vi "PLCtest.vi"(7 "Old VAL":bool[](array[boolean]), 10 "索引":i32, 11 "VISA资源名称":refnum<visa-resource-name>="COM2") -> (0 "错误输出":errorcluster)   [LabVIEW 2011]
uses:
  <vilib>/Instr/_visa.llb/VISA Configure Serial Port (Instr).vi
panel:
  in  "错误输入（无错误） 2":errorcluster caption="错误输入（无错误）"
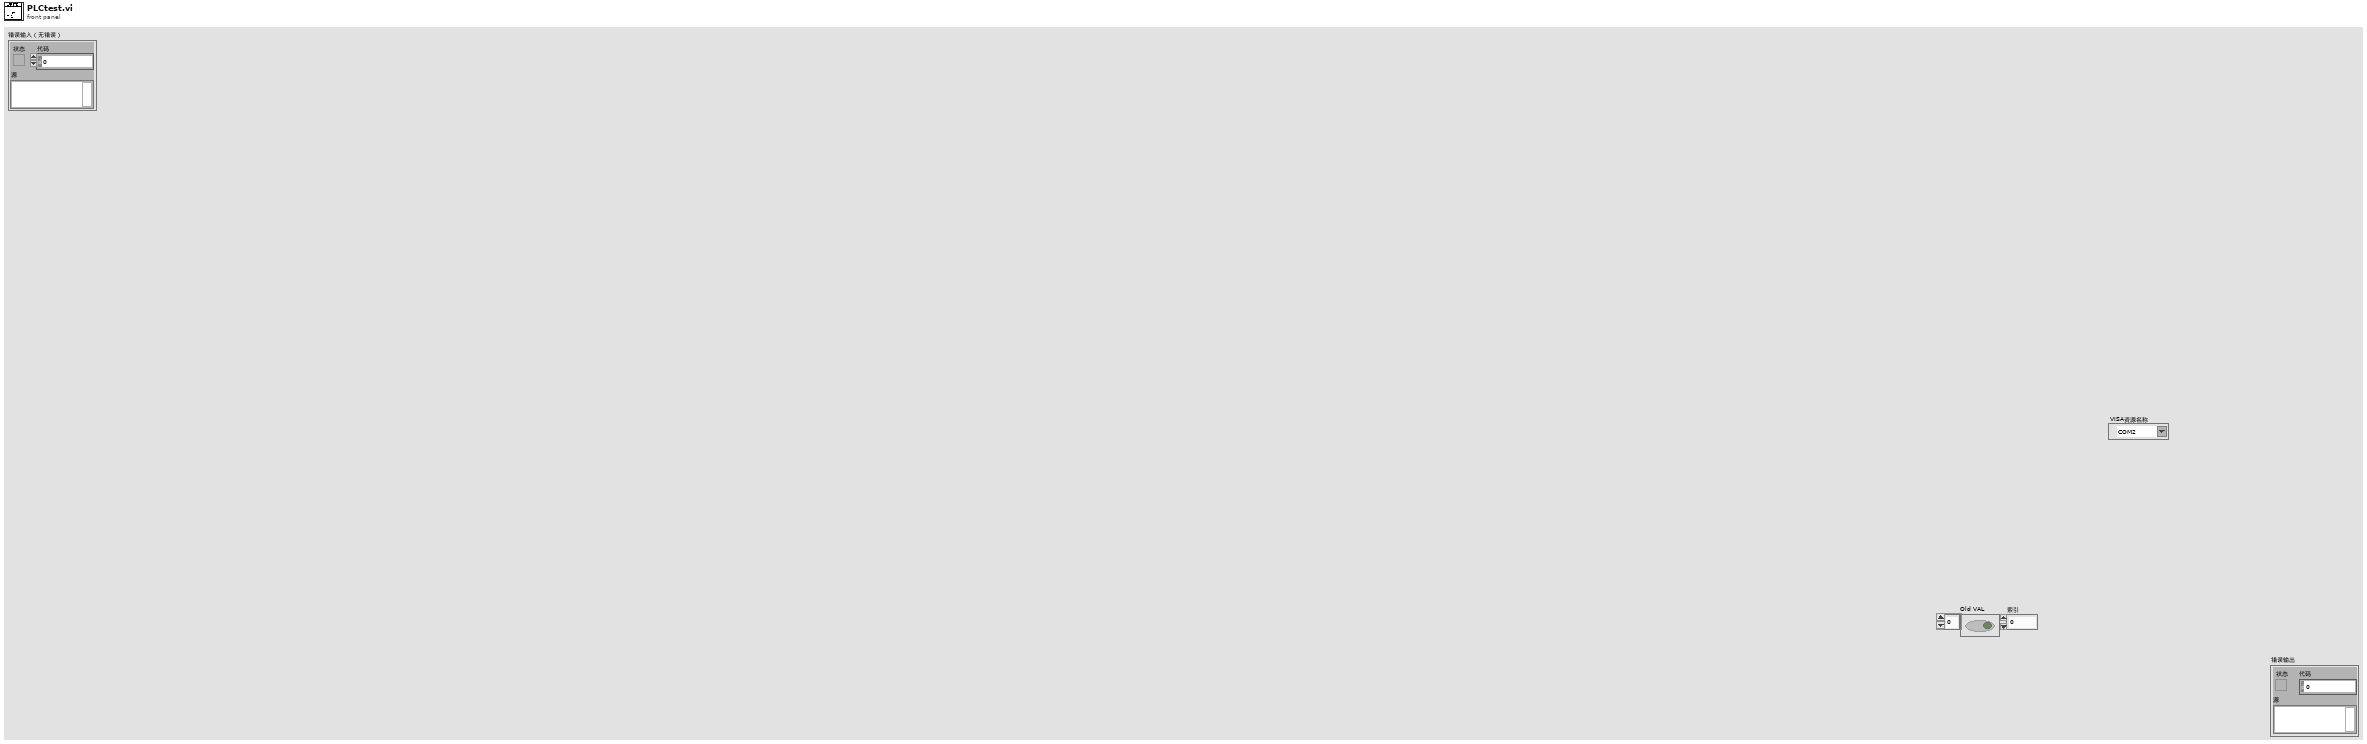
[diagram p1: front panel]
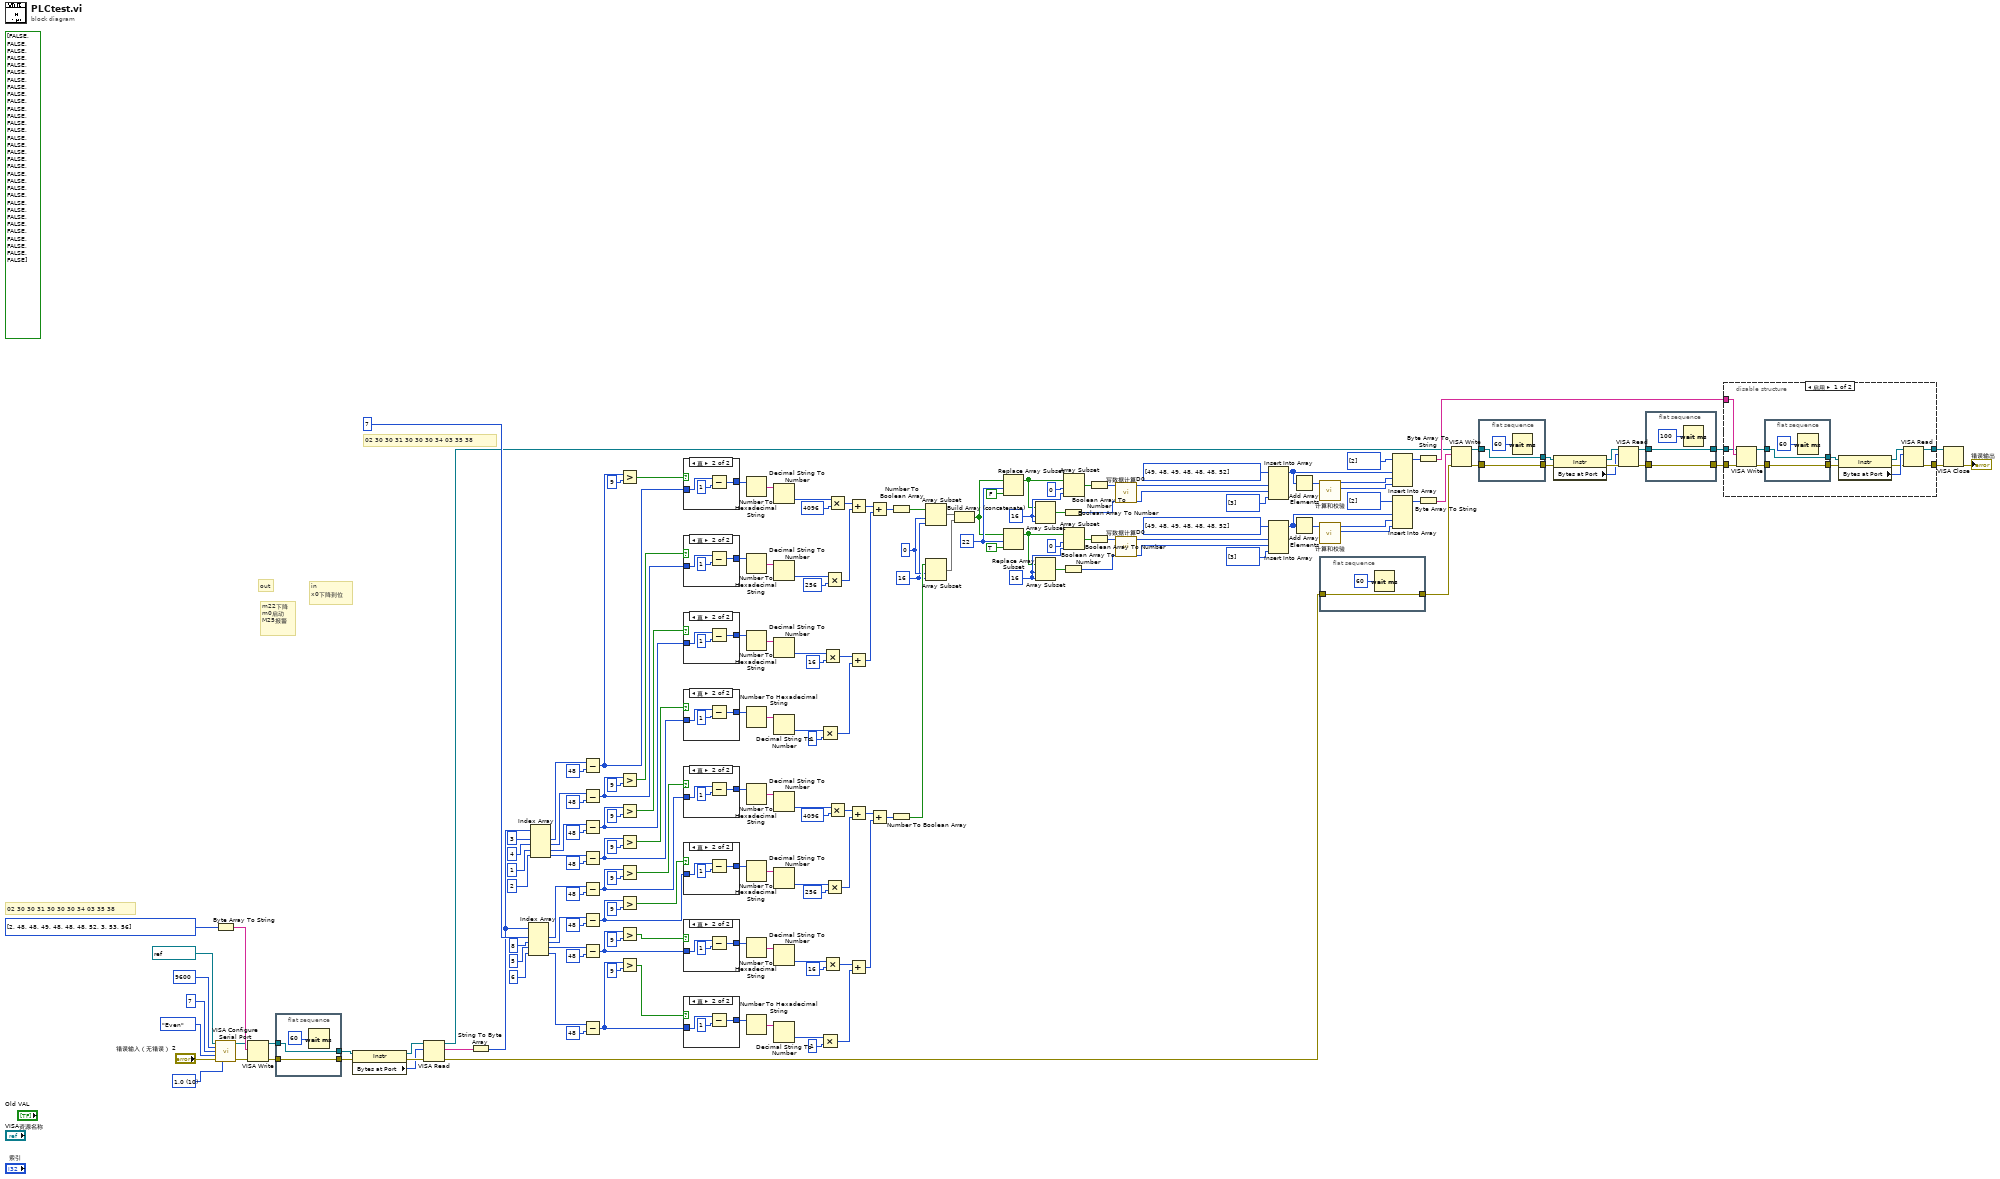
[diagram p0: block diagram]
diagram:
  w10 = u16 10 items=["1.0"=10, "1.5"=15, "2.0"=20] ("停止位")
  w15 = 16 ("长度")
  w16 = 0 ("索引")
  (unwired) bool[] [FALSE, FALSE, FALSE, FALSE, FALSE, FALSE, FALSE, FALSE, FALSE, FALSE, FALSE, FALSE, FALSE, FALSE, FALSE, FALSE, FALSE, FALSE, FALSE, FALSE, FALSE, FALSE, FALSE, FALSE, FALSE, FALSE, FALSE, FALSE, FALSE, FALSE, FALSE, FALSE] ("M 2")
  w124 = 22 ("索引")
  w149 = 16 ("长度")
  w155 = 16 ("长度")
  # "in\nx0下降到位"
  # "out"
  # "02 30 30 31 30 30 30 34 03 35 38"
  # "02 30 30 31 30 30 30 34 03 35 38"
  # "m22下降\nm0启动\nM25报警"
  n1 = Byte Array To String(unsigned byte array=u8[] [2, 48, 48, 49, 48, 48, 48, 52, 3, 53, 56] ("无符号字节数组")) -> (string=w121:string)
  n2 = call-poly "VISA Configure Serial Port"("VISA resource name"=refnum<visa-resource-name> "COM2" ("VISA资源名称"), "baud rate (9600)"=u32 9600 ("波特率"), "data bits (8)"=u16 7 ("数据位"), "parity (0:none)"=enum16{"None", "Odd", "Even", "Mark", "Space"}."Even" ("校验位"), "error in (no error)"="错误输入（无错误） 2", "stop bits (10: 1 bit)"=w10) -> ("VISA resource name out"=w5:refnum<visa-resource-name>, "error out"=w3:errorcluster)  [unwired: 8 in]
  n3 = VISA Write(VISA resource name=w5, write buffer=w121, error in (no error)=w3) -> (VISA resource name out=w122:refnum<visa-resource-name>, error out=w123:errorcluster)  [unwired: 1 out]
  n4 = flat-sequence {
    tunnel: w123 -> [w179]
    tunnel: [w179] -> w116
    tunnel: w122 -> [w178]
    tunnel: [w178] -> w117
    frame #0 {
      n5 = Wait (ms)(milliseconds to wait=u32 60 ("等待时间（毫秒）")) -> ()  [unwired: 1 out]
    }
  }
  n6 = property class="Instr"(reference=w117, error in=w116) -> (reference out=w120:refnum<visa-resource-name>, error out=w119:errorcluster, "Bytes at Port"=w118:u32)
  n7 = VISA Read(VISA resource name=w120, byte count=w118, error in (no error)=w119) -> (VISA resource name out=w11:refnum<visa-resource-name>, read buffer=w115:string, error out=w2:errorcluster)  [unwired: 1 out]
  n8 = String To Byte Array(string=w115) -> (unsigned byte array=w20:u8[])
  n9 = Index Array(array=w20, index #1=7 ("索引"), index #2=8 ("索引"), index #3=5 ("索引"), index #4=6 ("索引")) -> (element #1=w25:u8, element #2=w28:u8, element #3=w30:u8, element #4=w32:u8)
  n10 = Index Array(array=w20, index #1=3 ("索引"), index #2=4 ("索引"), index #3=1 ("索引"), index #4=2 ("索引")) -> (element #1=w110:u8, element #2=w107:u8, element #3=w105:u8, element #4=w103:u8)
  n11 = Subtract(x=w110, y=u8 48) -> (x-y=w91:u8)
  n12 = Subtract(x=w107, y=u8 48) -> (x-y=w94:u8)
  n13 = Subtract(x=w105, y=u8 48) -> (x-y=w97:u8)
  n14 = Subtract(x=w103, y=u8 48) -> (x-y=w101:u8)
  n15 = Subtract(x=w25, y=u8 48) -> (x-y=w44:u8)
  n16 = Subtract(x=w28, y=u8 48) -> (x-y=w41:u8)
  n17 = Subtract(x=w30, y=u8 48) -> (x-y=w38:u8)
  n18 = Subtract(x=w32, y=u8 48) -> (x-y=w34:u8)
  n19 = Greater?(x=w91, y=u8 9) -> (0:w93:bool)
  n20 = Greater?(x=w94, y=u8 9) -> (0:w95:bool)
  n21 = Greater?(x=w97, y=u8 9) -> (0:w99:bool)
  n22 = Greater?(x=w101, y=u8 9) -> (0:w100:bool)
  n23 = Greater?(x=w44, y=u8 9) -> (0:w42:bool)
  n24 = Greater?(x=w41, y=u8 9) -> (0:w40:bool)
  n25 = Greater?(x=w38, y=u8 9) -> (0:w36:bool)
  n26 = Greater?(x=w34, y=u8 9) -> (0:w35:bool)
  n27 = case shown="真" w93 {
    tunnel: w91 -> [w180 w183]
    tunnel: [w180 w181] -> w90
    frame False {
    }
    frame True {
      n28 = Subtract(x=w183, y=u8 1) -> (x-y=w181:u8)
    }
  }
  n29 = case shown="真" w95 {
    tunnel: w94 -> [w184 w187]
    tunnel: [w184 w185] -> w89
    frame False {
    }
    frame True {
      n30 = Subtract(x=w187, y=u8 1) -> (x-y=w185:u8)
    }
  }
  n31 = case shown="真" w99 {
    tunnel: w97 -> [w188 w191]
    tunnel: [w188 w189] -> w88
    frame False {
    }
    frame True {
      n32 = Subtract(x=w191, y=u8 1) -> (x-y=w189:u8)
    }
  }
  n33 = case shown="真" w100 {
    tunnel: w101 -> [w192 w195]
    tunnel: [w192 w193] -> w87
    frame False {
    }
    frame True {
      n34 = Subtract(x=w195, y=u8 1) -> (x-y=w193:u8)
    }
  }
  n35 = case shown="真" w42 {
    tunnel: w44 -> [w196 w199]
    tunnel: [w196 w197] -> w45
    frame False {
    }
    frame True {
      n36 = Subtract(x=w199, y=u8 1) -> (x-y=w197:u8)
    }
  }
  n37 = case shown="真" w40 {
    tunnel: w41 -> [w200 w203]
    tunnel: [w200 w201] -> w46
    frame False {
    }
    frame True {
      n38 = Subtract(x=w203, y=u8 1) -> (x-y=w201:u8)
    }
  }
  n39 = case shown="真" w36 {
    tunnel: w38 -> [w204 w207]
    tunnel: [w204 w205] -> w47
    frame False {
    }
    frame True {
      n40 = Subtract(x=w207, y=u8 1) -> (x-y=w205:u8)
    }
  }
  n41 = case shown="真" w35 {
    tunnel: w34 -> [w208 w211]
    tunnel: [w208 w209] -> w48
    frame False {
    }
    frame True {
      n42 = Subtract(x=w211, y=u8 1) -> (x-y=w209:u8)
    }
  }
  n43 = Number To Hexadecimal String(2:w90) -> (0:w86:string)  [unwired: 1 in]
  n44 = Number To Hexadecimal String(2:w89) -> (0:w85:string)  [unwired: 1 in]
  n45 = Number To Hexadecimal String(2:w88) -> (0:w84:string)  [unwired: 1 in]
  n46 = Number To Hexadecimal String(2:w87) -> (0:w83:string)  [unwired: 1 in]
  n47 = Number To Hexadecimal String(2:w45) -> (0:w49:string)  [unwired: 1 in]
  n48 = Number To Hexadecimal String(2:w46) -> (0:w50:string)  [unwired: 1 in]
  n49 = Number To Hexadecimal String(2:w47) -> (0:w51:string)  [unwired: 1 in]
  n50 = Number To Hexadecimal String(2:w48) -> (0:w52:string)  [unwired: 1 in]
  n51 = Decimal String To Number(string=w86) -> (number=w82:i32)  [unwired: 2 in, 1 out]
  n52 = Decimal String To Number(string=w85) -> (number=w81:i32)  [unwired: 2 in, 1 out]
  n53 = Decimal String To Number(string=w84) -> (number=w80:i32)  [unwired: 2 in, 1 out]
  n54 = Decimal String To Number(string=w83) -> (number=w79:i32)  [unwired: 2 in, 1 out]
  n55 = Decimal String To Number(string=w49) -> (number=w53:i32)  [unwired: 2 in, 1 out]
  n56 = Decimal String To Number(string=w50) -> (number=w54:i32)  [unwired: 2 in, 1 out]
  n57 = Decimal String To Number(string=w51) -> (number=w55:i32)  [unwired: 2 in, 1 out]
  n58 = Decimal String To Number(string=w52) -> (number=w56:i32)  [unwired: 2 in, 1 out]
  n59 = Multiply(x=w79, y=1) -> (x*y=w73:i32)
  n60 = Multiply(x=w56, y=1) -> (x*y=w62:i32)
  n61 = Multiply(x=w80, y=16) -> (x*y=w72:i32)
  n62 = Multiply(x=w55, y=16) -> (x*y=w63:i32)
  n63 = Multiply(x=w81, y=256) -> (x*y=w74:i32)
  n64 = Multiply(x=w54, y=256) -> (x*y=w61:i32)
  n65 = Multiply(x=w82, y=4096) -> (x*y=w69:i32)
  n66 = Multiply(x=w53, y=4096) -> (x*y=w66:i32)
  n67 = Add(x=w69, y=w74) -> (x+y=w70:i32)
  n68 = Add(x=w72, y=w73) -> (x+y=w71:i32)
  n69 = Add(x=w66, y=w61) -> (x+y=w65:i32)
  n70 = Add(x=w63, y=w62) -> (x+y=w64:i32)
  n71 = Add(x=w70, y=w71) -> (x+y=w68:i32)
  n72 = Add(x=w65, y=w64) -> (x+y=w67:i32)
  n73 = Number To Boolean Array(number=w68) -> (Boolean array=w17:bool[])
  n74 = Number To Boolean Array(number=w67) -> (Boolean array=w18:bool[])
  n75 = Array Subset(array=w17, index=w16, length=w15) -> (w13:bool[])
  n76 = Array Subset(array=w18, index=w16, length=w15) -> (w14:bool[])
  n77 = Build Array (concatenate)(w13, w14) -> (w12:bool[])
  n78 = Replace Array Subset(array=w12, new element=FALSE, index=w124) -> (w128:bool[])
  n79 = Replace Array Subset(array=w12, new element=TRUE ("Val"), index=w124) -> (w154:bool[])
  n80 = Array Subset(array=w128, index=w149, length=w149) -> (w151:bool[])
  n81 = Array Subset(array=w154, index=w155, length=w155) -> (w152:bool[])
  n82 = Boolean Array To Number(Boolean array=w151) -> (number=w147:u32)
  n83 = Boolean Array To Number(Boolean array=w152) -> (number=w157:u32)
  n84 = Array Subset(array=w128, index=0 ("索引"), length=w149) -> (w150:bool[])
  n85 = Array Subset(array=w154, index=0 ("索引"), length=w155) -> (w153:bool[])
  n86 = Boolean Array To Number(Boolean array=w150) -> (number=w146:u32)
  n87 = Boolean Array To Number(Boolean array=w153) -> (number=w158:u32)
  n88 = call "写数据计算D0.vi"("D0 2"=w147, "D0"=w146) -> ("数组 2"=w145:u32[], "数组"=w139:u32[])  [unwired: 8 in]
  n89 = call "写数据计算D0.vi"("D0 2"=w157, "D0"=w158) -> ("数组 2"=w159:u32[], "数组"=w165:u32[])  [unwired: 8 in]
  n90 = Insert Into Array(array=u16[] [49, 48, 49, 48, 48, 48, 52], new element #1=w139, new element #2=w145, new element #3=u16[] [3]) -> (w140:u16[])  [unwired: 1 in]
  n91 = Insert Into Array(array=u16[] [49, 48, 49, 48, 48, 48, 52], new element #1=w165, new element #2=w159, new element #3=u16[] [3]) -> (w164:u16[])  [unwired: 1 in]
  n92 = Add Array Elements(numeric array=w140) -> (sum=w143:u16)
  n93 = Add Array Elements(numeric array=w164) -> (sum=w161:u16)
  n94 = call "计算和校验.vi"("和"=w143) -> ("底"=w142:u32, "高"=w141:u32)  [unwired: 9 in]
  n95 = call "计算和校验.vi"("和"=w161) -> ("底"=w162:u32, "高"=w163:u32)  [unwired: 9 in]
  n96 = flat-sequence {
    tunnel: [w212] -> w1
    tunnel: w2 -> [w212]
    frame #0 {
      n97 = Wait (ms)(milliseconds to wait=u32 60 ("等待时间（毫秒）")) -> ()  [unwired: 1 out]
    }
  }
  n98 = Insert Into Array(array=u16[] [2], new element #1=w140, new element #2=w141, new element #3=w142) -> (w137:u16[])  [unwired: 1 in]
  n99 = Insert Into Array(array=u16[] [2], new element #1=w164, new element #2=w163, new element #3=w162) -> (w167:u16[])  [unwired: 1 in]
  n100 = Byte Array To String(unsigned byte array=w137) -> (string=w135:string)
  n101 = Byte Array To String(unsigned byte array=w167) -> (string=w174:string)
  n102 = VISA Write(VISA resource name=w11, write buffer=w174, error in (no error)=w1) -> (VISA resource name out=w175:refnum<visa-resource-name>, error out=w176:errorcluster)  [unwired: 1 out]
  n103 = flat-sequence {
    tunnel: w176 -> [w216]
    tunnel: [w216] -> w169
    tunnel: w175 -> [w215]
    tunnel: [w215] -> w170
    frame #0 {
      n104 = Wait (ms)(milliseconds to wait=u32 60 ("等待时间（毫秒）")) -> ()  [unwired: 1 out]
    }
  }
  n105 = property class="Instr"(reference=w170, error in=w169) -> (reference out=w173:refnum<visa-resource-name>, error out=w172:errorcluster, "Bytes at Port"=w171:u32)
  n106 = VISA Read(VISA resource name=w173, byte count=w171, error in (no error)=w172) -> (VISA resource name out=w134:refnum<visa-resource-name>, error out=w133:errorcluster)  [unwired: 2 out]
  n107 = flat-sequence {
    tunnel: w134 -> [w218]
    tunnel: w133 -> [w217]
    tunnel: [w218] -> w132
    tunnel: [w217] -> w131
    frame #0 {
      n108 = Wait (ms)(milliseconds to wait=u32 100 ("等待时间（毫秒）")) -> ()  [unwired: 1 out]
    }
  }
  n109 = disable-structure shown="启用" {
    disable-tunnel: w135 -> [w224 _]
    disable-tunnel: w132 -> [w223 w236]
    disable-tunnel: w131 -> [w222 w235]
    disable-tunnel: [w221 w236] -> w127
    disable-tunnel: [w220 w235] -> w126
    frame Enabled {
      n110 = VISA Write(VISA resource name=w223, write buffer=w224, error in (no error)=w222) -> (VISA resource name out=w226:refnum<visa-resource-name>, error out=w225:errorcluster)  [unwired: 1 out]
      n111 = flat-sequence {
        tunnel: w225 -> [w234]
        tunnel: [w234] -> w231
        tunnel: w226 -> [w233]
        tunnel: [w233] -> w230
        frame #0 {
          n112 = Wait (ms)(milliseconds to wait=u32 60 ("等待时间（毫秒）")) -> ()  [unwired: 1 out]
        }
      }
      n113 = property class="Instr"(reference=w230, error in=w231) -> (reference out=w227:refnum<visa-resource-name>, error out=w228:errorcluster, "Bytes at Port"=w229:u32)
      n114 = VISA Read(VISA resource name=w227, byte count=w229, error in (no error)=w228) -> (VISA resource name out=w221:refnum<visa-resource-name>, error out=w220:errorcluster)  [unwired: 2 out]
    }
    frame Disabled {
    }
  }
  n115 = VISA Close(VISA resource name=w127, error in (no error)=w126) -> (error out=→"错误输出":errorcluster)
